vi "Change_filter.vi"(8 "error in":errorcluster, 10 "filter number":string, 11 "VISA resource name":refnum<visa-resource-name>) -> (0 "error out":errorcluster, 3 "VISA resource name out":refnum<visa-resource-name>)   [LabVIEW 2018]
uses:
  <vilib>/Instr/_visa.llb/VISA Configure Serial Port (Instr).vi
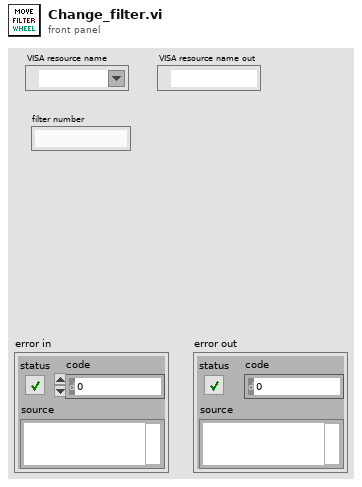
[diagram p1: front panel]
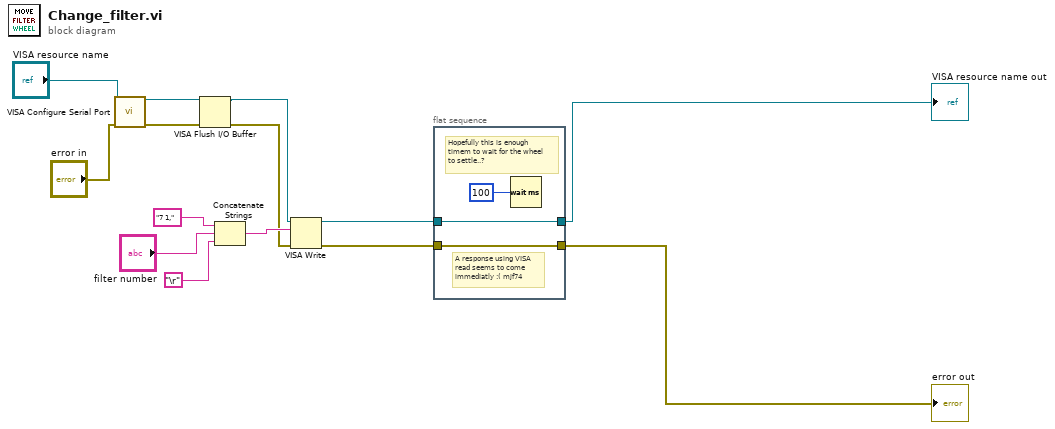
[diagram p0: block diagram]
diagram:
  n1 = call-poly "VISA Configure Serial Port"("VISA resource name"="VISA resource name", "error in (no error)"="error in") -> ("VISA resource name out"=w9:refnum<visa-resource-name>, "error out"=w10:errorcluster)  [unwired: 12 in]
  n2 = VISA Flush I/O Buffer(VISA resource name=w9, error in (no error)=w10) -> (VISA resource name out=w8:refnum<visa-resource-name>, error out=w7:errorcluster)  [unwired: 1 in]
  n3 = Concatenate Strings("7 1," ("string"), "filter number", "\r") -> (w14:string)
  n4 = VISA Write(VISA resource name=w8, write buffer=w14, error in (no error)=w7) -> (VISA resource name out=w2:refnum<visa-resource-name>, error out=w4:errorcluster)  [unwired: 1 out]
  n5 = flat-sequence {
    tunnel: [w17] -> w3
    tunnel: w4 -> [w17]
    tunnel: w2 -> [w15]
    tunnel: [w15] -> w1
    frame #0 {
      # "Hopefully this is enough \ntimem to wait for the wheel\nto settle..?"
      # "A response using VISA\nread seems to come \nimmediatly :( mjf74"
      n6 = Wait (ms)(milliseconds to wait=u32 100) -> ()  [unwired: 1 out]
    }
  }
  "error out" <- w3
  "VISA resource name out" <- w1
